vi "Setup per test.vi"(7 "Cluster":T5={"Queue Array"=[], "Queue Element"={"state"="", "data"=variant}, "System Event"=refnum, "System Event RefNum"=refnum, "Queue List"=[], "LPCA COM"="", "Rotating"=FALSE, "PrecorAI"="", "T_0 Index"=0, "Bar Graph X"=[], "Channels"=[], "Active Indicies"=[], "Active Channels"=[], "Sample Frequency"=0.0, "Ibrake Sweep"=[], "RPM Sweep"=[], "Load Sweep"=[], "Step Height Sweep"=[], "Range Sweep"=[], "A Counter"=0, "B Counter"=0, "C Counter"=0, "#A"=0, "#B"=0, "#C"=0, "Current RPM"=0.0, "Current Ibrake"=0, "Current Range"=0, "Current Step Height"=0, "Load Bank"=enum."OFF", "Cfg Cntrls"=[], "T_Monitor Indices"=[], "Thermal Limit"=0, "Thermal Resume"=0, "Timer Reset"=FALSE, "Stop Time"=0.0, "Autotest"=FALSE, "Pulsed RPM Capture"=FALSE, "Get Sample"=FALSE, "Last State"="", "Reset Timeout"=FALSE, "Ctrl Refs"={"Test Details"=refnum, "Save Config"=refnum, "Load Config"=refnum, "Path"=refnum, "Snapshot"=refnum, "SS#"=refnum, "Ibrake"=refnum, "RPM Target"=refnum, "Spin"=refnum, "Load Bank"=refnum, "Start Test"=refnum, "Pause Test"=refnum, "Load Sweep"=refnum, "RPM Sweep"=refnum, "Ibrake Sweep"=refnum, "Filters"=refnum, "Sample Frequency"=refnum, "Data Setup"=refnum, "Pause"=refnum, "Stop Time"=refnum, "S Period"=refnum, "Range"=refnum, "Step Height"=refnum, "Step Height Sweep"=refnum, "Range Sweep"=refnum, "Available Tests"=refnum, "RPM Graph"=refnum, "RPM Knob"=refnum, "FanMode"=refnum, "Fan Mode LED Array"=refnum, "Thermal Equilibrium"=refnum, "Data Display"=refnum, "LPCA Error"=refnum, "LPCA Ramp"=refnum, "LPCA Range"=refnum, "LPCA Resistance"=refnum, "Analyze Read"=refnum, "Console Select"=refnum, "Sub Panel"=refnum}, "Pulse Waveform"={"t0"=timestamp(0 s since 1904-01-01), "dt"=1.0, "Y"=[]}, "Snapshot"={"Test Details"="test", "Version"="test", "Date"=timestamp(3493915594.3018084 s since 1904-01-01), "Selected Test"="man", "Snapshot Number"=0, "Time"=timestamp(3493915602.7292905 s since 1904-01-01), "Ibrake Setpoint"="1", "RPM Setpoint"="20", "Range Setpoint"="", "Step Height Setpoint"="", "Load Bank Setpoint"="15", "Measurement Headers"="a,b,c,1,2,3", "Measurements"="1,2,3,4,5,6,7,8", "A"=0, "B"=0, "C"=0, "Raw Data"=[], "Available Tests"=enum."Manual", "Ibrake List"="", "RPM List"="", "Load Bank List"="", "Range List"="", "Step Height List"="", "FanMode Setpoint"=enum."Auto"}, "Sample Period"=0.0, "OverTemp"=FALSE, "Available Tests"=enum."Manual", "FanMode"=enum."Auto", "Fan Mode LED Array"=[FALSE, TRUE, FALSE], "Thermal\nEquilibrium "=FALSE, "Equilibrium Stop"=FALSE, "AvgDegChg"=[]} {"Snapshot"."Time" format="%<%H:%M:%S>T"; "Snapshot"."Date" format="%<%m/%d/%Y>T"}, 8 "error in (no error)":errorcluster, 9 "Label.Text":string, 10 "NewVal":T3, 11 "Enum in":refnum<vi>) -> (0 "error out":errorcluster, 1 "Man Disabled":T4(ring), 2 "Test Status":string, 3 "String":string, 4 "Graphic Display":T1, 5 "Man Enabled":T4(ring), 6 "Auto Test Controls":T2)   [LabVIEW 2017]
uses:
  Controls/Test TypeDef.ctl
  Code Library/Queue References Array.ctl
  Code Library/Queue Element.ctl
  Controls/Load Bank.ctl
  Controls/Available Tests.ctl
  Console Sim/Controls/Console Select.ctl
  Controls/Snapshot Typedef.ctl
  Controls/FanMode.ctl
  Controls/Auto Test Display.ctl
  Controls/Graphic Display.ctl
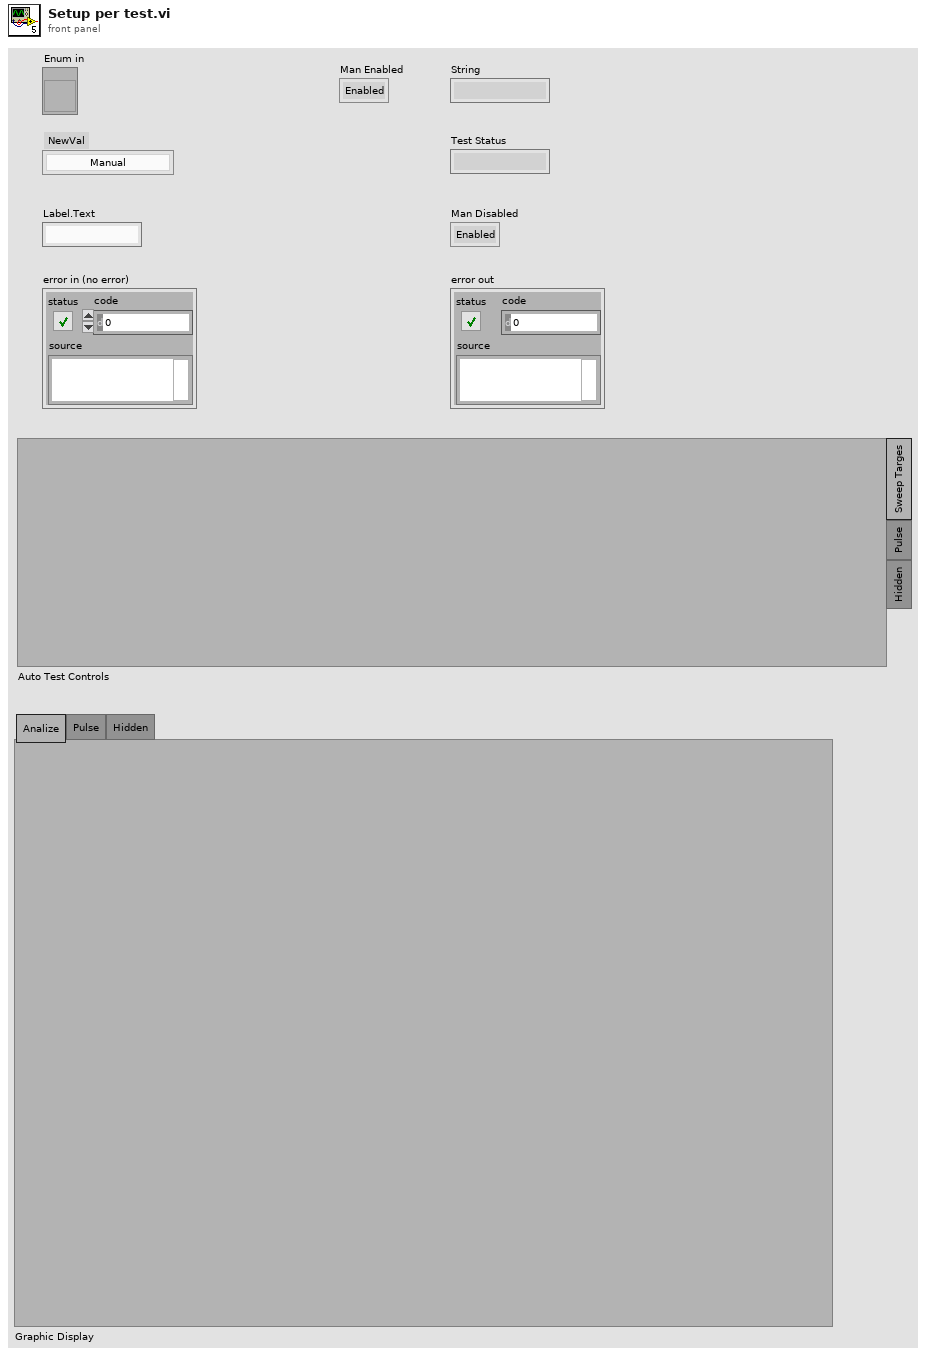
[diagram p1: front panel]
types:
  T1 = typedef "Graphic Display.ctl" = enum32{"Analize", "Pulse", "Hidden"}
  T2 = typedef "Auto Test Display.ctl" = enum32{"Sweep Targes", "Pulse", "Hidden"}
  T3 = typedef "Available Tests.ctl" = enum16{"Manual", "EFX Brake Torque", "Generator Torque", "EFX Brake Thermal", "Generator Thermal", "Pulsed RPM", "AMT Brake Torque", "Bike Brake Torque", "AMT Brake Thermal", "Bike Brake Thermal"}
  T4 = enum8{"Enabled", "Disabled", "Disabled and Grayed Out"}
  T5 = typedef "Test TypeDef.ctl" = cluster{"Queue Array":T6, "Queue Element":T7, "System Event":refnum<user-event>, "System Event RefNum":refnum<event-registration>, "Queue List":string[], "LPCA COM":refnum<visa-resource-name>, "Rotating":bool, "PrecorAI":refnum<k21>, "T_0 Index":i32, "Bar Graph X":i32[], "Channels":string[], "Active Indicies":i32[], "Active Channels":string[][], "Sample Frequency":dbl, "Ibrake Sweep":string[], "RPM Sweep":string[], "Load Sweep":string[], "Step Height Sweep":string[], "Range Sweep":string[], "A Counter":i32, "B Counter":i32, "C Counter":i32, "#A":i32, "#B":i32, "#C":i32, "Current RPM":dbl, "Current Ibrake":u32, "Current Range":u32, "Current Step Height":u32, "Load Bank":T8, "Cfg Cntrls":refnum<vi>[], "T_Monitor Indices":i32[], "Thermal Limit":i32, "Thermal Resume":i32, "Timer Reset":bool, "Stop Time":dbl, "Autotest":bool, "Pulsed RPM Capture":bool, "Get Sample":bool, "Last State":string, "Reset Timeout":bool, "Ctrl Refs":cluster{"Test Details":refnum<vi>, "Save Config":refnum<vi>, "Load Config":refnum<vi>, "Path":refnum<vi>, "Snapshot":refnum<vi>, "SS#":refnum<vi>, "Ibrake":refnum<vi>, "RPM Target":refnum<vi>, "Spin":refnum<vi>, "Load Bank":refnum<vi>, "Start Test":refnum<vi>, "Pause Test":refnum<vi>, "Load Sweep":refnum<vi>, "RPM Sweep":refnum<vi>, "Ibrake Sweep":refnum<vi>, "Filters":refnum<vi>, "Sample Frequency":refnum<vi>, "Data Setup":refnum<vi>, "Pause":refnum<vi>, "Stop Time":refnum<vi>, "S Period":refnum<vi>, "Range":refnum<vi>, "Step Height":refnum<vi>, "Step Height Sweep":refnum<vi>, "Range Sweep":refnum<vi>, "Available Tests":refnum<vi>, "RPM Graph":refnum<vi>, "RPM Knob":refnum<vi>, "FanMode":refnum<vi>, "Fan Mode LED Array":refnum<vi>, "Thermal Equilibrium":refnum<vi>, "Data Display":refnum<vi>, "LPCA Error":refnum<vi>, "LPCA Ramp":refnum<vi>, "LPCA Range":refnum<vi>, "LPCA Resistance":refnum<vi>, "Analyze Read":refnum<vi>, "Console Select":refnum<vi>, "Sub Panel":refnum<vi>}, "Pulse Waveform":waveform(dbl), "Snapshot":T9, "Sample Period":dbl, "OverTemp":bool, "Available Tests":T3, "FanMode":T10, "Fan Mode LED Array":bool[], "Thermal\nEquilibrium ":bool, "Equilibrium Stop":bool, "AvgDegChg":dbl[]}
  T6 = typedef "Queue References Array.ctl" = refnum<queue>[]
  T7 = typedef "Queue Element.ctl" = cluster{"state":string, "data":variant}
  T8 = typedef "Load Bank.ctl" = enum16{"OFF", "50", "25", "16.7", "12.5", "10.0", "8.3", "7.1", "6.3", "5.6", "5.0", "4.5", "4.2", "3.8", "3.6", "3.3", "3.1"}
  T9 = typedef "Snapshot Typedef.ctl" = cluster{"Test Details":string, "Version":string, "Date":timestamp, "Selected Test":string, "Snapshot Number":u16, "Time":timestamp, "Ibrake Setpoint":string, "RPM Setpoint":string, "Range Setpoint":string, "Step Height Setpoint":string, "Load Bank Setpoint":string, "Measurement Headers":string, "Measurements":string, "A":i32, "B":i32, "C":i32, "Raw Data":string[][], "Available Tests":T3, "Ibrake List":string, "RPM List":string, "Load Bank List":string, "Range List":string, "Step Height List":string, "FanMode Setpoint":T10}
  T10 = typedef "FanMode.ctl" = enum16{"On", "Off", "Auto"}
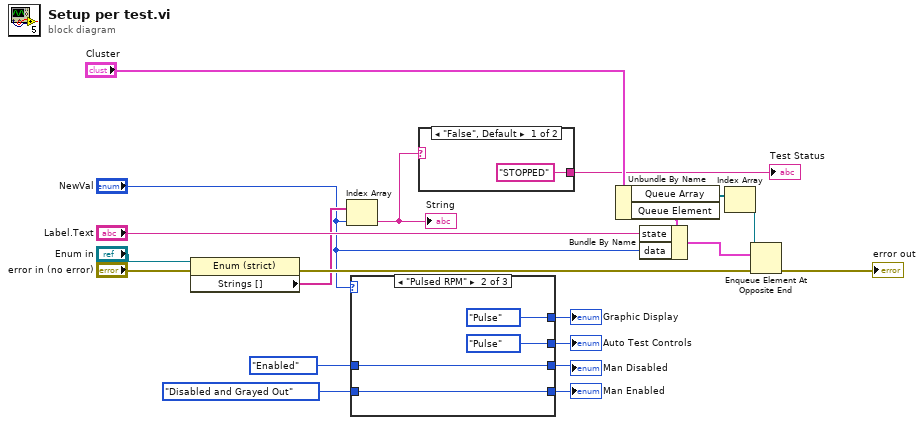
[diagram p0: block diagram]
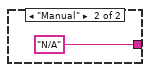
[diagram p2: hidden frame]
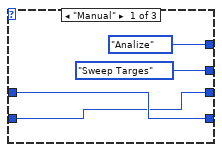
[diagram p3: hidden frame]
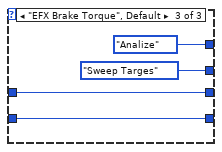
[diagram p4: hidden frame]
diagram:
  n1 = property class="Enum (strict)"(reference="Enum in", error in="error in (no error)") -> (error out=w7:errorcluster, "Strings []"=w5:string[])  [unwired: 1 out]
  n2 = Index Array(array=w5, index="NewVal") -> (element=w8:string)
  "String" <- w8
  n3 = case shown="\"Pulsed RPM\"" "NewVal" {
    tunnel: [w24 w28 w31] -> w10
    tunnel: T4."Enabled" ("Disabled") -> [w24 w27 w32]
    tunnel: T4."Disabled and Grayed Out" ("Disabled") -> [w23 w28 w31]
    tunnel: [w23 w27 w32] -> w20
    tunnel: [Graphic_Display."Analize" ("Graphic Display") Graphic_Display."Pulse" ("Graphic Display") Graphic_Display."Analize" ("Graphic Display")] -> w2
    tunnel: [Auto_Test_Display."Sweep Targes" ("Auto Test Controls") Auto_Test_Display."Pulse" ("Auto Test Controls") Auto_Test_Display."Sweep Targes" ("Auto Test Controls")] -> w1
    frame "Manual" {
    }
    frame "Pulsed RPM" {
    }
    frame "EFX Brake Torque", Default {
    }
  }
  "Man Disabled" <- w20
  "Man Enabled" <- w10
  "Auto Test Controls" <- w1
  "Graphic Display" <- w2
  n4 = case shown="\"False\", Default" w8 {
    tunnel: ["STOPPED" ("Test Status") "N/A" ("Test Status")] -> w9
    frame "False", Default {
    }
    frame "Manual" {
    }
  }
  "Test Status" <- w9
  n5 = Unbundle By Name("Cluster") -> ("Queue Array"=w13:T6, "Queue Element"=w15:T7)
  n6 = Bundle By Name(cluster=w15, "state"="Label.Text", "data"="NewVal") -> (w16:T7)
  n7 = Index Array(array=w13) -> (element=w14:refnum<queue>)  [unwired: 1 in]
  n8 = Enqueue Element At Opposite End(queue=w14, element=w16, error in (no error)=w7) -> (error out=→"error out":errorcluster)  [unwired: 1 in, 2 out]
